vi "Build Cal Array.vi"(0 "TextIn":string, 5 "NewPage":bool, 7 "PageNum":i32, 9 "PageTitle":string, 11 "CalDataIn":T1(array[cluster]) {"ChlFactor" format="%.3f"; "ChlZero" format="%.3f"}) -> (4 "TextOut":string, 8 "Err":bool, 10 "Done":bool, 15 "CalDataOut":T1(array[cluster]) {"ChlFactor" format="%.3f"; "ChlZero" format="%.3f"})   [LabVIEW 2013]
panel:
  out "Chl_Config":u16
  out "Chl_Factor":sgl format="%.2f"
  out "Chl_Zero":sgl format="%.2f"
  out "Chl_Units":string
  out "Chl_Desc":string
  out "Chl_Num":string
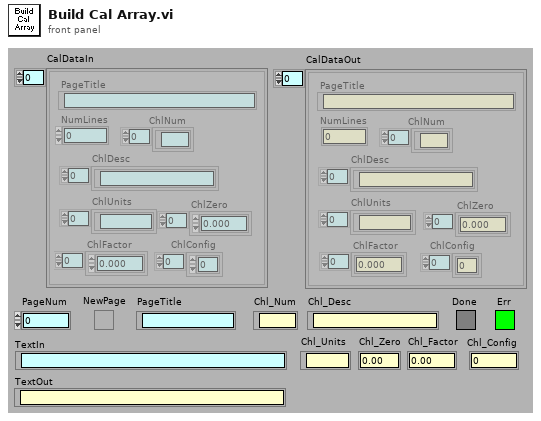
[diagram p1: front panel]
types:
  T1 = cluster{"PageTitle":string, "NumLines":i32, "ChlNum":string[], "ChlDesc":string[], "ChlUnits":string[], "ChlZero":sgl[], "ChlFactor":sgl[], "ChlConfig":u16[]}[]
  T2 = cluster{"PageTitle":string, "NumLines":i32, "ChlNum":string[], "ChlDesc":string[], "ChlUnits":string[], "ChlZero":sgl[], "ChlFactor":sgl[], "ChlConfig":u16[]}
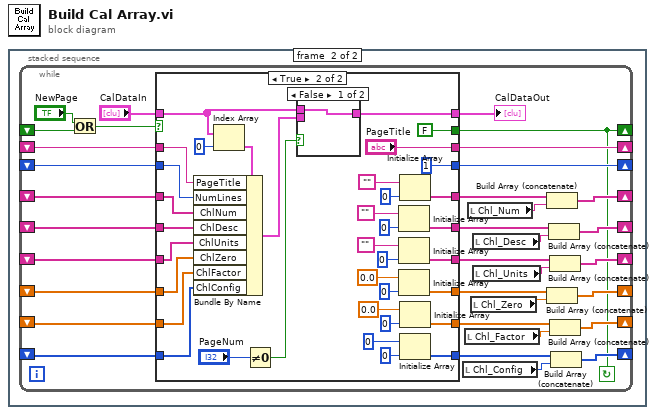
[diagram p0: block diagram]
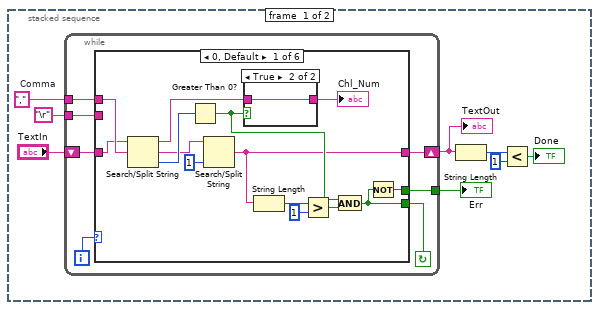
[diagram p2: hidden frame]
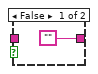
[diagram p3: hidden frame]
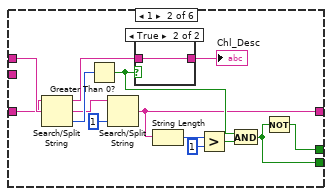
[diagram p4: hidden frame]
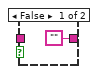
[diagram p5: hidden frame]
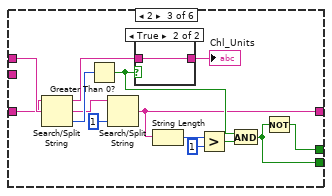
[diagram p6: hidden frame]
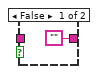
[diagram p7: hidden frame]
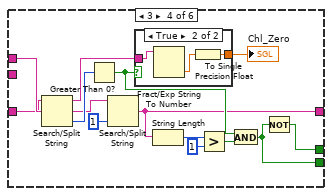
[diagram p8: hidden frame]
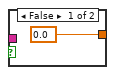
[diagram p9: hidden frame]
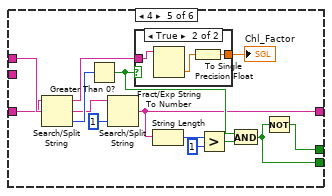
[diagram p10: hidden frame]
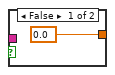
[diagram p11: hidden frame]
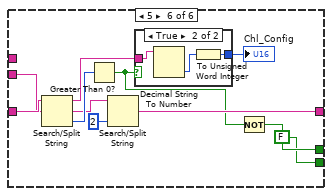
[diagram p12: hidden frame]
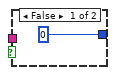
[diagram p13: hidden frame]
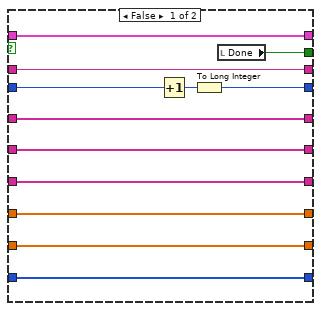
[diagram p14: hidden frame]
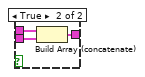
[diagram p15: hidden frame]
diagram:
  n1 = stacked-sequence {
    frame #0 {
      w7 = ","  # Comma
      n2 = while {
        tunnel: [w9] -> w1
        tunnel: "\r" -> [w12]
        tunnel: w7 -> [w13]
        shift-left: "TextIn" -> [w14]
        shift-right: [w11] -> w2
        i -> [w15]
        stop <- w10 continue-if-true
        n3 = case shown="0, Default" w15 {
          tunnel: w14 -> [w28 w44 w60 w76 w94 w110]
          tunnel: w13 -> [w29 w45 w61 w77 w95 _]
          tunnel: w12 -> [_ _ _ _ _ w102]
          tunnel: [w18 w35 w51 w67 w85 w105] -> w11
          tunnel: [w16 w34 w50 w66 w84 FALSE] -> w10
          tunnel: [w17 w33 w49 w65 w83 w104] -> w9
          frame 0, Default {
            n4 = Search/Split String(string=w28, search string/char (-)=w29) -> (substring before match=w24:string, match + rest of string=w25:string, offset of match=w27:i32)  [unwired: 1 in]
            n5 = Greater Than 0?(x=w27) -> (x > 0?=w20:bool)
            n6 = Search/Split String(string=w25, offset (0)=1) -> (match + rest of string=w18:string)  [unwired: 1 in, 2 out]
            n7 = case shown="True" w20 {
              tunnel: ["" w31] -> w19
              tunnel: w24 -> [_ w31]
              frame False {
              }
              frame True {
              }
            }
            "Chl_Num" <- w19
            n8 = String Length(string=w18) -> (length=w23:i32)
            n9 = Greater?(x=w23, y=1) -> (0:w21:bool)
            n10 = And(x=w20, y=w21) -> (x .and. y?=w16:bool)
            n11 = Not(x=w16) -> (.not. x?=w17:bool)
          }
          frame 1 {
            n12 = Search/Split String(string=w44, search string/char (-)=w45) -> (substring before match=w40:string, match + rest of string=w41:string, offset of match=w43:i32)  [unwired: 1 in]
            n13 = Greater Than 0?(x=w43) -> (x > 0?=w36:bool)
            n14 = Search/Split String(string=w41, offset (0)=1) -> (match + rest of string=w35:string)  [unwired: 1 in, 2 out]
            n15 = case shown="True" w36 {
              tunnel: ["" w47] -> w32
              tunnel: w40 -> [_ w47]
              frame False {
              }
              frame True {
              }
            }
            "Chl_Desc" <- w32
            n16 = String Length(string=w35) -> (length=w39:i32)
            n17 = Greater?(x=w39, y=1) -> (0:w37:bool)
            n18 = And(x=w36, y=w37) -> (x .and. y?=w34:bool)
            n19 = Not(x=w34) -> (.not. x?=w33:bool)
          }
          frame 2 {
            n20 = Search/Split String(string=w60, search string/char (-)=w61) -> (substring before match=w56:string, match + rest of string=w57:string, offset of match=w59:i32)  [unwired: 1 in]
            n21 = Greater Than 0?(x=w59) -> (x > 0?=w52:bool)
            n22 = Search/Split String(string=w57, offset (0)=1) -> (match + rest of string=w51:string)  [unwired: 1 in, 2 out]
            n23 = case shown="True" w52 {
              tunnel: ["" w63] -> w48
              tunnel: w56 -> [_ w63]
              frame False {
              }
              frame True {
              }
            }
            "Chl_Units" <- w48
            n24 = String Length(string=w51) -> (length=w55:i32)
            n25 = Greater?(x=w55, y=1) -> (0:w53:bool)
            n26 = And(x=w52, y=w53) -> (x .and. y?=w50:bool)
            n27 = Not(x=w50) -> (.not. x?=w49:bool)
          }
          frame 3 {
            n28 = Search/Split String(string=w76, search string/char (-)=w77) -> (substring before match=w72:string, match + rest of string=w73:string, offset of match=w75:i32)  [unwired: 1 in]
            n29 = Greater Than 0?(x=w75) -> (x > 0?=w68:bool)
            n30 = Search/Split String(string=w73, offset (0)=1) -> (match + rest of string=w67:string)  [unwired: 1 in, 2 out]
            n31 = case shown="True" w68 {
              tunnel: w72 -> [_ w81]
              tunnel: [sgl 0.0 w80] -> w64
              frame False {
              }
              frame True {
                n32 = Fract/Exp String To Number(string=w81) -> (number=w79:dbl)  [unwired: 3 in, 1 out]
                n33 = To Single Precision Float(number=w79) -> (single precision float=w80:sgl)
              }
            }
            "Chl_Zero" <- w64
            n34 = String Length(string=w67) -> (length=w71:i32)
            n35 = Greater?(x=w71, y=1) -> (0:w69:bool)
            n36 = And(x=w68, y=w69) -> (x .and. y?=w66:bool)
            n37 = Not(x=w66) -> (.not. x?=w65:bool)
          }
          frame 4 {
            n38 = Search/Split String(string=w94, search string/char (-)=w95) -> (substring before match=w90:string, match + rest of string=w91:string, offset of match=w93:i32)  [unwired: 1 in]
            n39 = Greater Than 0?(x=w93) -> (x > 0?=w86:bool)
            n40 = Search/Split String(string=w91, offset (0)=1) -> (match + rest of string=w85:string)  [unwired: 1 in, 2 out]
            n41 = case shown="True" w86 {
              tunnel: w90 -> [_ w99]
              tunnel: [sgl 0.0 w98] -> w82
              frame False {
              }
              frame True {
                n42 = Fract/Exp String To Number(string=w99) -> (number=w97:dbl)  [unwired: 3 in, 1 out]
                n43 = To Single Precision Float(number=w97) -> (single precision float=w98:sgl)
              }
            }
            "Chl_Factor" <- w82
            n44 = String Length(string=w85) -> (length=w89:i32)
            n45 = Greater?(x=w89, y=1) -> (0:w87:bool)
            n46 = And(x=w86, y=w87) -> (x .and. y?=w84:bool)
            n47 = Not(x=w84) -> (.not. x?=w83:bool)
          }
          frame 5 {
            n48 = Search/Split String(string=w110, search string/char (-)=w102) -> (substring before match=w106:string, match + rest of string=w107:string, offset of match=w109:i32)  [unwired: 1 in]
            n49 = Greater Than 0?(x=w109) -> (x > 0?=w100:bool)
            n50 = Search/Split String(string=w107, offset (0)=2) -> (match + rest of string=w105:string)  [unwired: 1 in, 2 out]
            n51 = case shown="True" w100 {
              tunnel: w106 -> [_ w114]
              tunnel: [u16 0 w113] -> w103
              frame False {
              }
              frame True {
                n52 = Decimal String To Number(string=w114) -> (number=w112:i32)  [unwired: 2 in, 1 out]
                n53 = To Unsigned Word Integer(number=w112) -> (unsigned 16bit integer=w113:u16)
              }
            }
            "Chl_Config" <- w103
            n54 = Not(x=w100) -> (.not. x?=w104:bool)
          }
        }
      }
      "Err" <- w1
      "TextOut" <- w2
      n55 = String Length(string=w2) -> (length=w4:i32)
      n56 = Less?(x=w4, y=1) -> (x < y?=→"Done":bool)
    }
    frame #1 {
      n57 = while {
        shift-left: _ -> [w116]
        shift-right: [w115] -> _
        shift-left: _ -> [w139]
        shift-right: [w140] -> _
        shift-left: _ -> [w117]
        shift-right: [w129] -> _
        shift-left: _ -> [w118]
        shift-right: [w130] -> _
        shift-left: _ -> [w119]
        shift-right: [w131] -> _
        shift-left: _ -> [w120]
        shift-right: [w132] -> _
        shift-left: _ -> [w121]
        shift-right: [w133] -> _
        shift-left: _ -> [w122]
        shift-right: [w134] -> _
        shift-left: _ -> [w148]
        shift-right: [w141] -> _
        stop <- w115 continue-if-true
        n58 = Or(x="NewPage", y=w116) -> (x .or. y?=w138:bool)
        n59 = case shown="True" w138 {
          tunnel: w148 -> [w159 w174]
          tunnel: [w157 1] -> w141
          tunnel: [w160 w193] -> w128
          tunnel: w122 -> [w160 w173]
          tunnel: [w156 w190] -> w127
          tunnel: w121 -> [w156 w172]
          tunnel: [w155 w187] -> w126
          tunnel: w120 -> [w155 w171]
          tunnel: w119 -> [w154 w170]
          tunnel: [w153 w182] -> w124
          tunnel: w118 -> [w153 w169]
          tunnel: [w152 w179] -> w123
          tunnel: w117 -> [w152 w168]
          tunnel: [w151 "PageTitle"] -> w140
          tunnel: w139 -> [w151 w175]
          tunnel: "CalDataIn" -> [w150 w166]
          tunnel: [w150 w165] -> w135
          tunnel: [w154 w162] -> w125
          tunnel: [w149 FALSE] -> w115
          frame False {
            n60 = Increment(x=w159) -> (x+1=w158:i32)
            n61 = To Long Integer(number=w158) -> (32bit integer=w157:i32)
            n62 = local read "Done"() -> (w149:bool)
          }
          frame True {
            n63 = Index Array(array=w166, index=0 ("Index")) -> (element=w177:T2)
            n64 = Bundle By Name(cluster=w177, "PageTitle"=w175, "NumLines"=w174, "ChlNum"=w173, "ChlDesc"=w172, "ChlUnits"=w171, "ChlZero"=w170, "ChlFactor"=w169, "ChlConfig"=w168) -> (w167:T2)
            n65 = Not Equal To 0?(x="PageNum") -> (x != 0?=w163:bool)
            n66 = case shown="False" w163 {
              tunnel: w167 -> [_ w200]
              tunnel: w166 -> [w197 w199]
              tunnel: [w197 w198] -> w165
              frame False {
              }
              frame True {
                n67 = Build Array (concatenate)(w199, w200) -> (w198:T1)
              }
            }
            n68 = Initialize Array("", 0 ("Dimension Size")) -> (w190:string[])
            n69 = Initialize Array("", 0 ("Dimension Size")) -> (w187:string[])
            n70 = Initialize Array(sgl 0.0, 0 ("Dimension Size")) -> (w162:sgl[])
            n71 = Initialize Array("", 0 ("Dimension Size")) -> (w193:string[])
            n72 = Initialize Array(sgl 0.0, 0 ("Dimension Size")) -> (w182:sgl[])
            n73 = Initialize Array(u16 0, 0 ("Dimension Size")) -> (w179:u16[])
          }
        }
        "CalDataOut" <- w135
        n74 = local read "Chl_Config"() -> (w142:u16)
        n75 = local read "Chl_Factor"() -> (w143:sgl)
        n76 = local read "Chl_Num"() -> (w147:string)
        n77 = local read "Chl_Zero"() -> (w144:sgl)
        n78 = local read "Chl_Desc"() -> (w146:string)
        n79 = local read "Chl_Units"() -> (w145:string)
        n80 = Build Array (concatenate)(w128, w147) -> (w134:string[])
        n81 = Build Array (concatenate)(w125, w144) -> (w131:sgl[])
        n82 = Build Array (concatenate)(w127, w146) -> (w133:string[])
        n83 = Build Array (concatenate)(w126, w145) -> (w132:string[])
        n84 = Build Array (concatenate)(w124, w143) -> (w130:sgl[])
        n85 = Build Array (concatenate)(w123, w142) -> (w129:u16[])
      }
    }
  }
